vi "read TBM configuration.vi"(8 "error in":errorcluster, 11 "module editor node in":refnum<class "module editor node.lvclass">) -> (0 "error out":errorcluster, 2 "configuration":refnum<class "TBM configuration.lvclass">, 3 "module editor node out":refnum<class "module editor node.lvclass">)   [LabVIEW 2013, in "PL Framework Configuration Tool.lvlib" / "module editor node.lvclass"]
uses:
  module editor node.lvclass
  <vilib>/NI/Tag Bus Module Framework/root configuration/TBM configuration.lvclass
  <vilib>/NI/Tag Bus Module Framework/module configuration/TBM module configuration.lvclass
  <vilib>/NI/Tag Bus Module Framework/root configuration/TBM configuration.lvclass/TBM configuration.ctl
  TBM Configuration Node/TBM Configuration Node.lvclass
  <vilib>/NI/Tag Bus Module Framework/root configuration/create GUID.vi
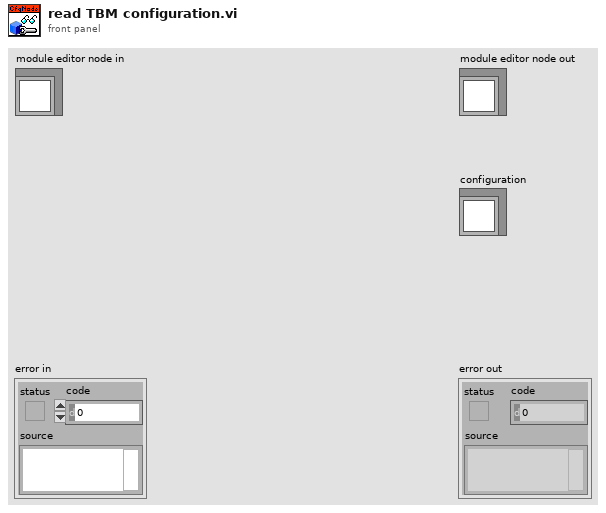
[diagram p1: front panel]
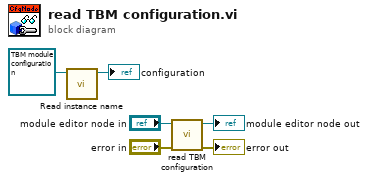
[diagram p0: block diagram]
diagram:
  n1 = call <vilib>:"Read instance name.vi"("configuration in"=refnum<class "TBM module configuration.lvclass"> refnum ("module configuration in")) -> ("configuration out"=→"configuration":refnum<class "TBM module configuration.lvclass">)  [unwired: 8 in, 2 out]
  n2 = call-parent "read TBM configuration.vi"("error in"="error in", "TBM Configuration Node in"="module editor node in") -> ("error out"=→"error out":errorcluster, "TBM Configuration Node out"=→"module editor node out":refnum<class "module editor node.lvclass">)  [unwired: 7 in, 1 out]
